vi "Brocadcast Models&Views.vi"(8 "error in (no error)":errorcluster, 11 "MVVM Abstruct Controller in":refnum<class "MVVM Abstruct Controller.lvclass">) -> (0 "error out":errorcluster, 3 "MVVM Abstruct Controller out":refnum<class "MVVM Abstruct Controller.lvclass">)   [LabVIEW 2020, in "MMVVM Framework.lvlib" / "MVVM Abstruct Controller.lvlib" / "MVVM Abstruct Controller.lvclass"]
uses:
  MVVM Abstruct Controller.lvclass
  Enqueues Data/Enqueues Data.lvclass
  MVVM Abstruct Controller.lvclass/MVVM Abstruct Controller.ctl
  Enqueues Data/Enqueues Data.lvclass/Enqueues Data.ctl
  Model&View Interface Messages/Brocast Data Msg/Brocast Data Msg.lvclass/Brocast Data Msg.ctl
  <vilib>/ActorFramework/Message Enqueuer/Message Enqueuer.lvclass/Message Enqueuer.ctl
  Enqueues Data/Accessors/Write ActorMap.vi
  <vilib>/ActorFramework/Message Enqueuer/Enqueue.vi
  Model&View Interface Messages/Brocast Data Msg/Brocast Data Msg.lvclass
  C:/Program Files (x86)/National Instruments/LabVIEW 2020/vi.lib/ActorFramework/Message/Message.lvclass
  <vilib>/ActorFramework/Message Priority Queue/Priority Enqueue.vi
  ActorMap/ActorMap.lvclass
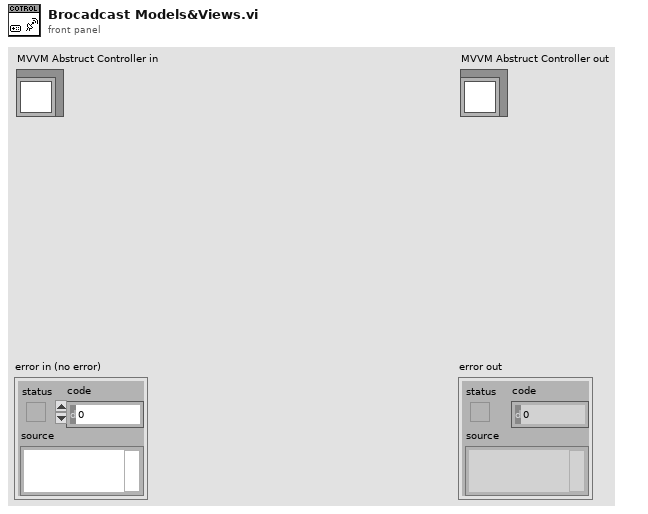
[diagram p1: front panel]
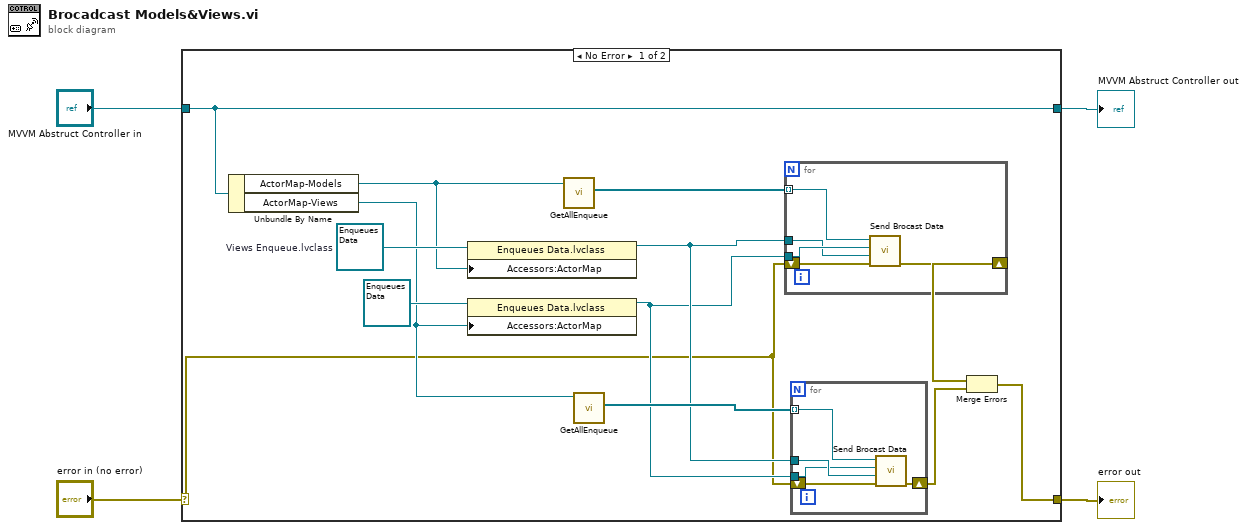
[diagram p0: block diagram]
diagram:
  n1 = case shown="No Error" "error in (no error)" {
    selector: "error in (no error)" -> [w8 w29]
    tunnel: [w5 w29] -> w3
    tunnel: [w17 w28] -> w1
    tunnel: "MVVM Abstruct Controller in" -> [w17 w28]
    frame No Error {
      w15 = refnum<class "Enqueues Data.lvclass"> refnum  # Views Enqueue.lvclass
      n2 = Unbundle By Name(w17) -> ("ActorMap-Models"=w14:refnum<class "ActorMap.lvclass">, "ActorMap-Views"=w12:refnum<class "ActorMap.lvclass">)
      n3 = property class="Enqueues Data.lvclass"(reference=w15, "Accessors:ActorMap"=w14) -> (reference out=w10:refnum<class "Enqueues Data.lvclass">)  [unwired: 1 in, 1 out]
      n4 = property class="Enqueues Data.lvclass"(reference=refnum<class "Enqueues Data.lvclass"> refnum ("Views Enqueue.lvclass"), "Accessors:ActorMap"=w12) -> (reference out=w9:refnum<class "Enqueues Data.lvclass">)  [unwired: 1 in, 1 out]
      n5 = call "GetAllEnqueue.vi"("ActorMap in"=w14) -> ("Enqueues"=w16:refnum<class "Message Enqueuer.lvclass">[])  [unwired: 7 in, 3 out]
      n6 = call "GetAllEnqueue.vi"("ActorMap in"=w12) -> ("Enqueues"=w11:refnum<class "Message Enqueuer.lvclass">[])  [unwired: 7 in, 3 out]
      n7 = for {
        tunnel: w16 -> [w27] mode=indexing
        tunnel: w10 -> [w23]
        tunnel: w9 -> [w24]
        shift-right: [w26] -> w7
        shift-left: w8 -> [w25]
        n8 = call "Send Brocast Data.vi"("error in (no error)"=w25, "Models Enqueue.lvclass"=w23, "Views Enqueue.lvclass"=w24, "Message Enqueuer"=w27) -> ("error out"=w26:errorcluster)  [unwired: 6 in, 1 out]
      }
      n9 = for {
        tunnel: w11 -> [w22] mode=indexing
        tunnel: w10 -> [w19]
        tunnel: w9 -> [w18]
        shift-right: [w21] -> w6
        shift-left: w8 -> [w20]
        n10 = call "Send Brocast Data.vi"("error in (no error)"=w20, "Models Enqueue.lvclass"=w19, "Views Enqueue.lvclass"=w18, "Message Enqueuer"=w22) -> ("error out"=w21:errorcluster)  [unwired: 6 in, 1 out]
      }
      n11 = Merge Errors(w7, w6) -> (w5:errorcluster)
    }
    frame Error {
    }
  }
  "error out" <- w3
  "MVVM Abstruct Controller out" <- w1
